vi "sub_UART.vi"(0 "Señal_1":dbl, 1 "Señal_2":dbl, 2 "Señal_3":dbl, 3 "Señal 4":dbl, 4 "Señal 5":dbl) -> (7 "US_3 3":string, 8 "Trama de envio":string, 9 "US_3 2":string, 10 "US_1":string, 11 "Sensor 5":dbl, 12 "US_2":string, 13 "Sensor 4":dbl, 14 "Sensor_1":dbl, 15 "Sensor_2":dbl, 16 "Trama Recibida":string, 17 "Sensor_3":dbl, 18 "US_3":string)   [LabVIEW 2019]
uses:
  <vilib>/myRIO/Instrument Drivers/Onboard IO/UART/typedef/VISA Configuration.ctl
  <vilib>/Instr/_visa.llb/VISA Configure Serial Port (Instr).vi
  <vilib>/myRIO/Express VI/Onboard IO/UART/UART Express VI.xnode
  <vilib>/myRIO/Instrument Drivers/Onboard IO/UART/UART.lvlib
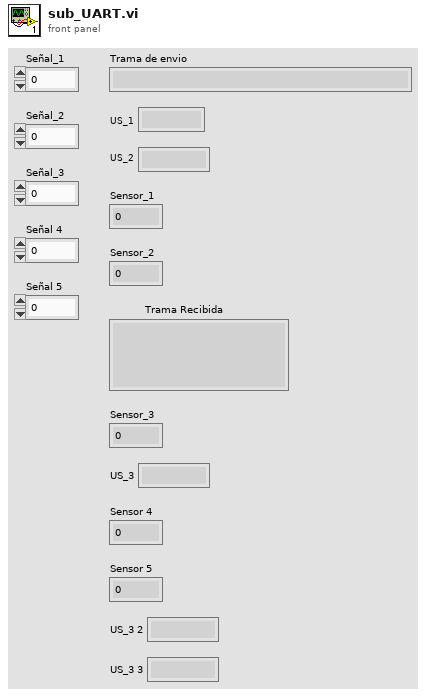
[diagram p1: front panel]
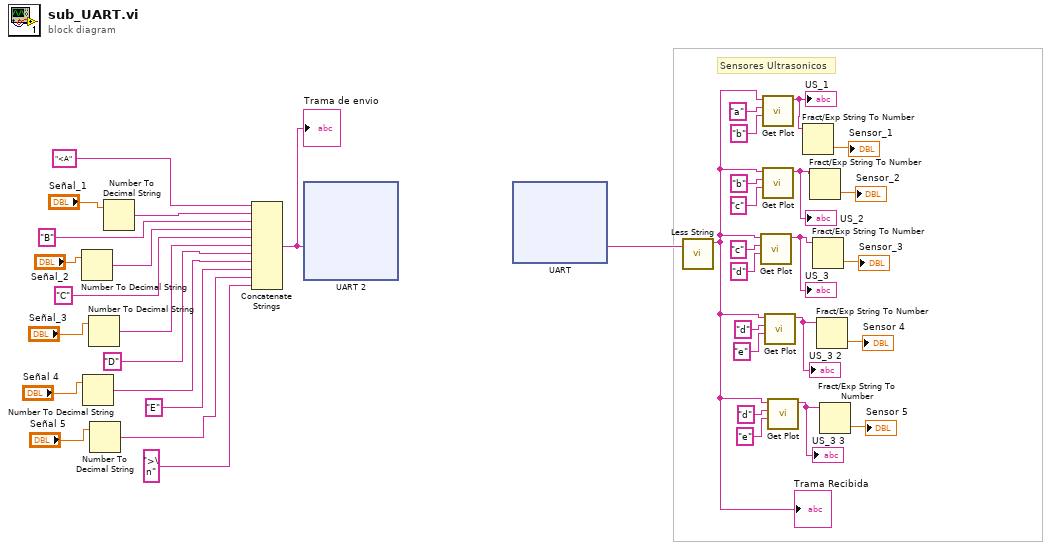
[diagram p0: block diagram]
diagram:
  # "Sensores Ultrasonicos"
  n1 = Number To Decimal String(number="Señal_2") -> (decimal integer string=w16:string)  [unwired: 1 in]
  n2 = Number To Decimal String(number="Señal 4") -> (decimal integer string=w27:string)  [unwired: 1 in]
  n3 = Number To Decimal String(number="Señal_3") -> (decimal integer string=w18:string)  [unwired: 1 in]
  n4 = Number To Decimal String(number="Señal 5") -> (decimal integer string=w29:string)  [unwired: 1 in]
  n5 = Number To Decimal String(number="Señal_1") -> (decimal integer string=w14:string)  [unwired: 1 in]
  n6 = Concatenate Strings("<A" ("string"), w14, "B" ("string"), w16, "C" ("string"), w18, "D" ("string"), w27, "E" ("string"), w29, ">\n" ("string")) -> (w23:string)
  "Trama de envio" <- w23
  n7 = xnode "UART 2"("Characters to Write"=w23) -> ()  [unwired: 1 in, 2 out]
  n8 = xnode "UART"() -> ("Characters Read"=w13:string)  [unwired: 1 in, 1 out]
  n9 = call "Less String.vi"("Input String"=w13) -> ("Out String"=w39:string)  [unwired: 10 in]
  "Trama Recibida" <- w39
  n10 = call "Get Plot.vi"("Stop"="d", "Start"="c", "Input String"=w39) -> ("Out String"=w12:string)  [unwired: 8 in]
  "US_3" <- w12
  n11 = call "Get Plot.vi"("Stop"="b", "Start"="a", "Input String"=w39) -> ("Out String"=w7:string)  [unwired: 8 in]
  "US_1" <- w7
  n12 = call "Get Plot.vi"("Stop"="c", "Start"="b", "Input String"=w39) -> ("Out String"=w11:string)  [unwired: 8 in]
  "US_2" <- w11
  n13 = call "Get Plot.vi"("Stop"="e", "Start"="d", "Input String"=w39) -> ("Out String"=w34:string)  [unwired: 8 in]
  "US_3 2" <- w34
  n14 = call "Get Plot.vi"("Stop"="e", "Start"="d", "Input String"=w39) -> ("Out String"=w38:string)  [unwired: 8 in]
  "US_3 3" <- w38
  n15 = Fract/Exp String To Number(string=w7) -> (number=→"Sensor_1":dbl)  [unwired: 3 in, 1 out]
  n16 = Fract/Exp String To Number(string=w11) -> (number=→"Sensor_2":dbl)  [unwired: 3 in, 1 out]
  n17 = Fract/Exp String To Number(string=w12) -> (number=→"Sensor_3":dbl)  [unwired: 3 in, 1 out]
  n18 = Fract/Exp String To Number(string=w34) -> (number=→"Sensor 4":dbl)  [unwired: 3 in, 1 out]
  n19 = Fract/Exp String To Number(string=w38) -> (number=→"Sensor 5":dbl)  [unwired: 3 in, 1 out]
